vi "ScatProps.vi"() -> ()   [LabVIEW 2022 SP3]
uses:
  <vilib>/Utility/file.llb/Write To Spreadsheet File (DBL).vi
panel:
  in  "Case Constant\n(See Context Help)":bool
  out "midband":cluster{dbl[], sgl[]}(graph)
  in  "con":dbl=1.0 format="%.2f"
  out "intercept":cluster{dbl[], sgl[]}(graph)
  out "slope":cluster{dbl[], sgl[]}(graph)
  in  "Calc type":enum32{"find spec params", "fixed size"}(tab)
  in  "stop radius mm":dbl=0.125 format="%.2f"
  in  "start radius mm":dbl=0.005 format="%.2f"
  in  "fixed radius (mm)":dbl=1.0 format="%.2f"
  in  "stop freq (MHz)":dbl=50.0 format="%.2f"
  in  "start freq (MHz)":dbl=10.0 format="%.2f"
  in  "fixed B":dbl=1.0 format="%.2f"
  in  "Data System params":T1={"sample freq (MHz)"=0.0, "focal length (mm)"=50.8, "aperature radius (mm)"=4.5, "pts in window"=64.0} {"pts in window" format="%.2f"; "aperature radius (mm)" format="%.2f"; "focal length (mm)" format="%.2f"; "sample freq (MHz)" format="%.2f"}
  in  "material props":T2={"sound speed mm/micros"=1.54, "particle Z"=2.0, "host Zo"=1.0, "scatterer"=0} {"scatterer" items=["isotropic", "cylindrical", "planar"]; "host Zo" format="%.2f"; "particle Z" format="%.2f"; "sound speed mm/micros" format="%.2f"}
  in  "Tranducer Info":T3 {"bandwidth" format="%.2f"; "center freq" format="%.2f"; "start freq" format="%.2f"}
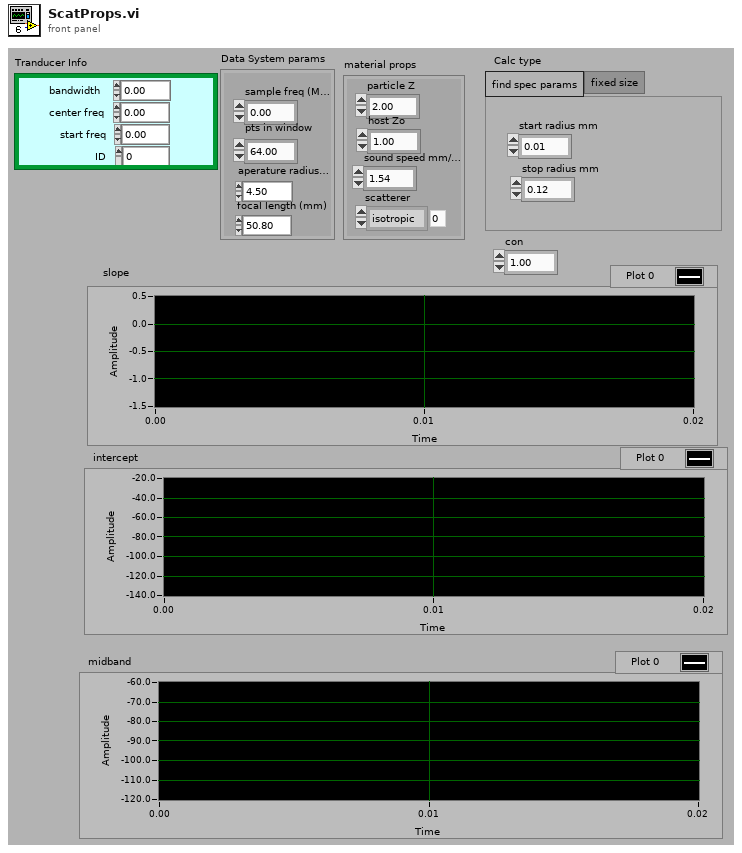
[diagram p1: front panel]
types:
  T1 = cluster{"sample freq (MHz)":dbl, "focal length (mm)":sgl, "aperature radius (mm)":sgl, "pts in window":dbl}
  T2 = cluster{"sound speed mm/micros":dbl, "particle Z":dbl, "host Zo":dbl, "scatterer":i32}
  T3 = cluster{"bandwidth":sgl, "center freq":sgl, "start freq":sgl, "ID":i32}
  T4 = cluster{"midband":sgl, "slope":sgl, "intercept":sgl}
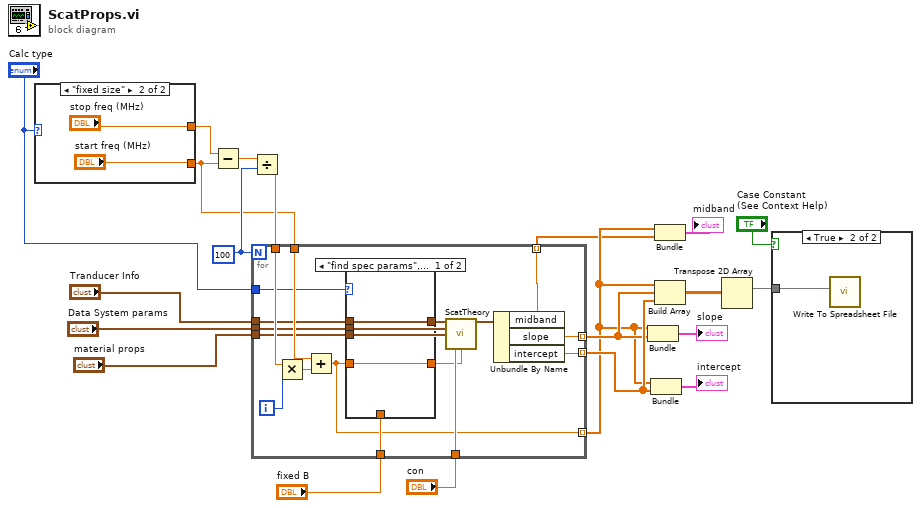
[diagram p0: block diagram]
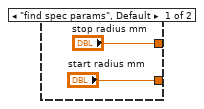
[diagram p3: hidden frame]
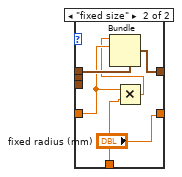
[diagram p4: hidden frame]
diagram:
  w15 = 100
  n1 = case shown="\"fixed size\"" "Calc type" {
    tunnel: ["stop radius mm" "stop freq (MHz)"] -> w17
    tunnel: ["start radius mm" "start freq (MHz)"] -> w11
    frame "find spec params", Default {
    }
    frame "fixed size" {
    }
  }
  n2 = Subtract(x=w17, y=w11) -> (x-y=w16:dbl)
  n3 = Divide(x=w16, y=w15) -> (x/y=w12:dbl)
  n4 = for {
    N: w15 -> [_]
    tunnel: "Tranducer Info" -> [w33]
    tunnel: "Data System params" -> [w30]
    tunnel: "material props" -> [w29]
    tunnel: "con" -> [w42]
    tunnel: [w40] -> w4 mode=indexing
    tunnel: [w36] -> w8 mode=indexing
    tunnel: w12 -> [w38]
    tunnel: w11 -> [w35]
    tunnel: "Calc type" -> [w31]
    tunnel: "fixed B" -> [w28]
    tunnel: [w27] -> w3 mode=indexing
    tunnel: [w26] -> w2 mode=indexing
    i -> [w39]
    n5 = Multiply(x=w38, y=w39) -> (x*y=w37:dbl)
    n6 = Add(x=w35, y=w37) -> (x+y=w27:dbl)
    n7 = case shown="\"find spec params\", Default" w31 {
      tunnel: [w44 "fixed radius (mm)"] -> w34
      tunnel: w27 -> [w44 w46]
      tunnel: [w43 w48] -> w32
      tunnel: w33 -> [w43 w49]
      tunnel: w30 -> [_ _]
      tunnel: w29 -> [_ _]
      tunnel: w28 -> [_ w47]
      frame "find spec params", Default {
      }
      frame "fixed size" {
        n8 = Multiply(x=w46, y=w47) -> (x*y=w45:dbl)
        n9 = Bundle(cluster=w49, "bandwidth"=w45, "center freq"=w46) -> (w48:T3)  [unwired: 2 out]
      }
    }
    n10 = call "ScatTheory.vi"("Tranducer Info"=w32, "Data System params"=w30, "material props"=w29, "con (part/cc)"=w42, "radius (mm)"=w34) -> ("spectral params"=w41:T4)  [unwired: 3 in, 7 out]
    n11 = Unbundle By Name(w41) -> ("midband"=w26:sgl, "slope"=w40:sgl, "intercept"=w36:sgl)
  }
  n12 = Bundle(w3, w4) -> (→"slope":cluster{dbl[], sgl[]})  [unwired: 1 out]
  n13 = Bundle(w3, w8) -> (→"intercept":cluster{dbl[], sgl[]})  [unwired: 1 out]
  n14 = Bundle(w3, w2) -> (→"midband":cluster{dbl[], sgl[]})  [unwired: 1 out]
  n15 = Build Array(w3, w4, w8) -> (w7:dbl[][])
  n16 = Transpose 2D Array(2D array=w7) -> (transposed array=w6:dbl[][])
  n17 = case shown="True" "Case Constant\n(See Context Help)" {
    tunnel: w6 -> [_ w51]
    frame False {
    }
    frame True {
      n18 = call-poly <vilib>:"Write To Spreadsheet File.vi"("2D data"=w51) -> ()  [unwired: 5 in, 3 out]
    }
  }
